vi "GetMSGName.vi"(11 "Popup Msg in":refnum<class "Popup Msg.lvclass">) -> (2 "NAME":string, 3 "Popup Msg out":refnum<class "Popup Msg.lvclass">)   [LabVIEW 2020, in "Test-Client.lvlib" / "Popup Msg.lvclass"]
uses:
  Popup Msg.lvclass
panel:
  # "e"
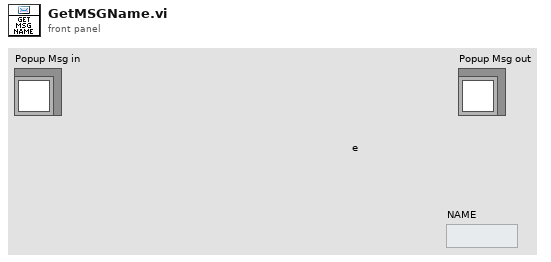
[diagram p1: front panel]
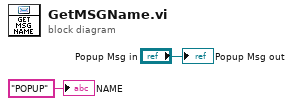
[diagram p0: block diagram]
diagram:
  "Popup Msg out" <- "Popup Msg in"
  "NAME" <- "POPUP" ("NAME")
